vi "DataType_to_String.vi"(4 "data type":T1) -> (1 "data type string":string)   [LabVIEW 2016, in "PyLVi.lvlib" / "PyLVi.lvclass"]
uses:
  PyLVi.lvclass
  Controls/DataType.ctl
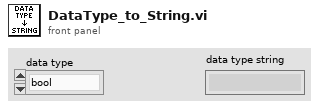
[diagram p1: front panel]
types:
  T1 = typedef "PyLVi.lvlib/PyLVi.lvclass/DataType.ctl" = enum16{"bool", "string", "int16", "int32", "float32", "float64", "complex128"}
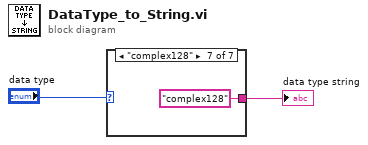
[diagram p0: block diagram]
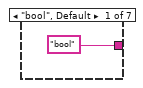
[diagram p2: hidden frame]
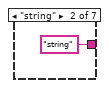
[diagram p3: hidden frame]
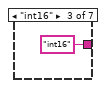
[diagram p4: hidden frame]
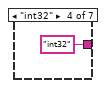
[diagram p5: hidden frame]
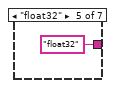
[diagram p6: hidden frame]
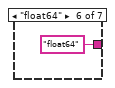
[diagram p7: hidden frame]
diagram:
  n1 = case shown="\"complex128\"" "data type" {
    tunnel: ["bool" ("data type string") "string" ("data type string") "int16" ("data type string") "int32" ("data type string") "float32" ("data type string") "float64" ("data type string") "complex128" ("data type string")] -> w1
    frame "bool", Default {
    }
    frame "string" {
    }
    frame "int16" {
    }
    frame "int32" {
    }
    frame "float32" {
    }
    frame "float64" {
    }
    frame "complex128" {
    }
  }
  "data type string" <- w1
